vi "Read data and open write session on first call.vi"(8 "error in (no error)":errorcluster, 11 "RT State Data in":T1) -> (0 "error out":errorcluster, 3 "RT State Data out":T1)   [LabVIEW 2013, in "Waveforms Generation Custom Device.lvlib"]
uses:
  Waveforms Generation Custom Device.lvlib
  RT state data.ctl
  <vilib>/NI Veristand/Custom Device API/Waveform Data Reference.ctl
  <vilib>/NI Veristand/Custom Device API/Custom Device API.lvlib
  <vilib>/NI Veristand/Custom Device Waveform API/Multiple Waveforms Write (DBL)/Multiple Waveforms Write (DBL).lvclass
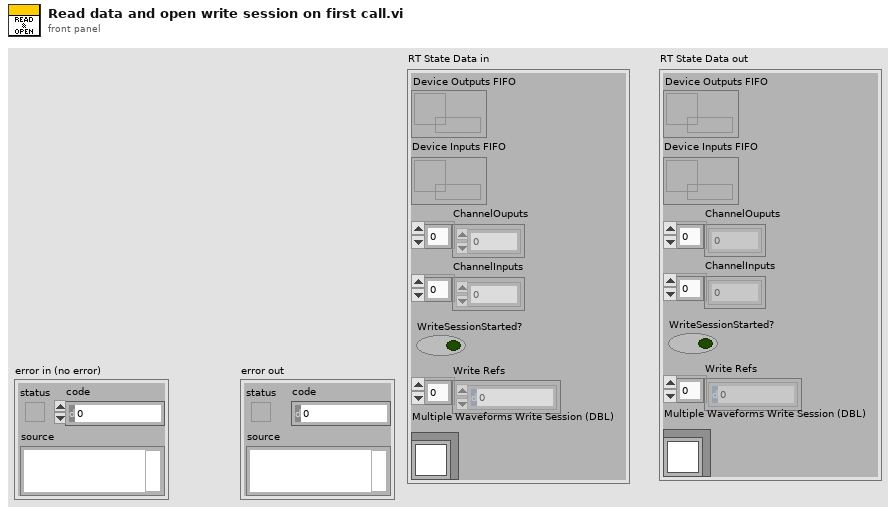
[diagram p1: front panel]
types:
  T1 = typedef "Waveforms Generation Custom Device.lvlib/RT state data.ctl" = cluster{"Device Outputs FIFO":refnum<k33>, "Device Inputs FIFO":refnum<k33>, "ChannelOuputs":dbl[], "ChannelInputs":dbl[], "WriteSessionStarted?":bool, "Write Refs":T2[], "Multiple Waveforms Write Session (DBL)":refnum<class "Multiple Waveforms Write (DBL).lvclass">}
  T2 = typedef "Custom Device API.lvlib/Waveform Data Reference.ctl" = i32
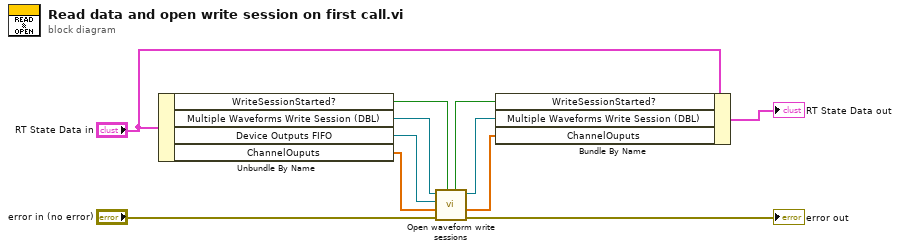
[diagram p0: block diagram]
diagram:
  n1 = Unbundle By Name("RT State Data in") -> ("WriteSessionStarted?"=w11:bool, "Multiple Waveforms Write Session (DBL)"=w5:refnum<class "Multiple Waveforms Write (DBL).lvclass">, "Device Outputs FIFO"=w3:refnum<k33>, "ChannelOuputs"=w2:dbl[])
  n2 = call "Open waveform write sessions.vi"("Already opened?"=w11, "error in (no error)"="error in (no error)", "ChannelOuputs In"=w2, "Device Outputs FIFO"=w3, "Multiple Waveforms Write Session (DBL)"=w5) -> ("error out"=→"error out":errorcluster, "ChannelOuputs Out"=w1:dbl[], "Multiple Waveforms Write Session (DBL)"=w4:refnum<class "Multiple Waveforms Write (DBL).lvclass">, "Opened"=w9:bool)  [unwired: 3 in]
  n3 = Bundle By Name(cluster="RT State Data in", "WriteSessionStarted?"=w9, "Multiple Waveforms Write Session (DBL)"=w4, "ChannelOuputs"=w1) -> (→"RT State Data out":T1)
